vi "HAILO_Main_3d.vi"() -> ()   [LabVIEW 2016]
doc: "This example performs writes and reads on a serial port, as directed by the user. You can press the Write and Read buttons, and change the Read Count, while the example is running.\n\nThe parameters set for the serial port must match the parameters of the connected instrument or device. In this example, the Read Count parameter specifies the number of bytes that the serial port reads. If there were more bytes at the port than the specified number, those bytes would not be read. If there were less bytes at the port than the specified number, you would receive a timeout error.\n\nThis example expands upon the flow control options for XON and XOFF, allowing the user to choose those control characters. Also, the user can enable or disable a termination character. Some devices require a termination character in order to identify the end of command strings. Some devices send a termination character to signify the end of data to be read. This example shows how you can end the Read operation once a termination character is detected in the buffer and/or append a termination character at the end of the Write data."
uses:
  <vilib>/ptbypt/NI_PtbyPt.lvlib
panel:
  out "Stop 3D":bool
  out "Connection Status":u16(ring) items=["Connecting....", "BT Connected", "Disconnected"]
  in  "Tab Control":T1(tab)
  out "Channel":u16
  in  "Device Name":string="HAILO_Watch"
  in  "F Shear":dbl[](array[numeric])=[0.1, 0.1, 0.1, 0.1]
  in  "dT desired (ms)":u32=20
  in  "3d Display dT":i32=40
  in  "Enable  3D":bool
  in  "Camera Controller":enum16{"None", "Spherical", "Flying"}(ring)=enum."Spherical"
  in  "Rendering Destination":enum16{"3D Window", "3D Off"}(ring)=enum."3D Off"
  in  "3D Display":bool
  out "Sensor Output":dbl[](array[numeric])
  out "read buffer":string
  out "Sensor Nodes Returned":i32=384
  out "Sensor Readings":i16[][](array[numeric])=[[-533, -111, 239], [-402, 166, 184], [-184, 154, 29], [-106, 74, 11], [-532, -109, 246], [-398, 164, 175], [-205, 152, 32], [-119, 65, 9], [-529, -110, 242], [-408, 166, 184], [-198, 158, 27], [-108, 61, 6], [-539, -106, 240], [-407, 158, 183], [-191, 156, 28], [-113, 73, 15], [816, -260, 842], [539, 512, 512], [156, 425, 83], [13, 142, -72], [816, -262, 840], [528, 520, 512], [162, 425, 83], [13, 137, -84], [809, -260, 840], [538, 520, 504], [162, 432, 72], [13, 136, -84], [809, -260, 846], [538, 508, 512], [158, 435, 72], [19, 136, -79], [346, -168, 14], [287, -68, 19], [161, -34, 4], [70, -44, -7], [345, -191, 19], [279, -40, 8], [167, -16, 12], [72, -23, 2], [341, -190, 17], [285, -46, 9], [149, -15, 6], [54, -40, -2], [375, -201, 19], [282, -51, 10], [135, -37, 6], [81, -57, -12], [-80, -193, -48], [-73, -136, -12], [-5, -122, -31], [-19, -118, -17], [-118, -187, -48], [-73, -115, -22], [1, -113, -27], [-20, -111, -8], [-99, -184, -40], [-62, -145, -17], [0, -113, -37], [-7, -117, -15], [-126, -184, -50], [-72, -115, -14], [-4, -114, -25], [-29, -116, -14]]
  out "Packet OK?":bool=TRUE
  out "Packets Recieved":i32
  out "dT (ms)":dbl
  out "Shear Force":T2(graph)
  out "Normal Force":T3(graph)
  out "Time":u32=427420
  in  "Zero?":bool
  in  "Stop":bool
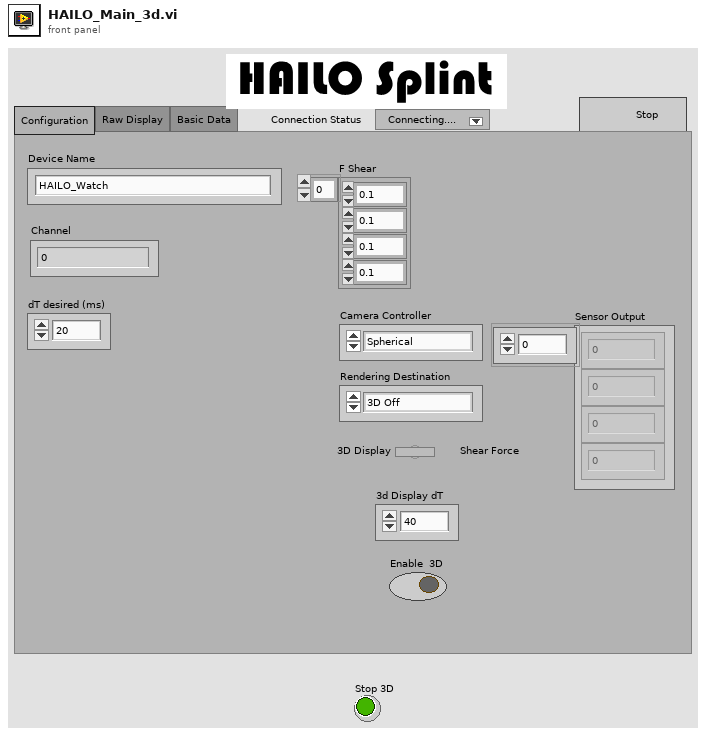
[diagram p1: front panel]
types:
  T1 = enum32{"Configuration", "Raw Display", "Basic Data"}
  T2 = cluster{"F Shear[0]":dbl, "F Shear[1]":dbl, "F Shear[2]":dbl, "F Shear[3]":dbl}
  T3 = cluster{"F Normal[0]":dbl, "F Normal[1]":dbl, "F Normal[2]":dbl, "F Normal[3]":dbl}
  T4 = cluster{"channel":u16, "uuid":string, "service name":string, "service description":string}[]
  T5 = cluster{"channel":u16, "uuid":string, "service name":string, "service description":string}
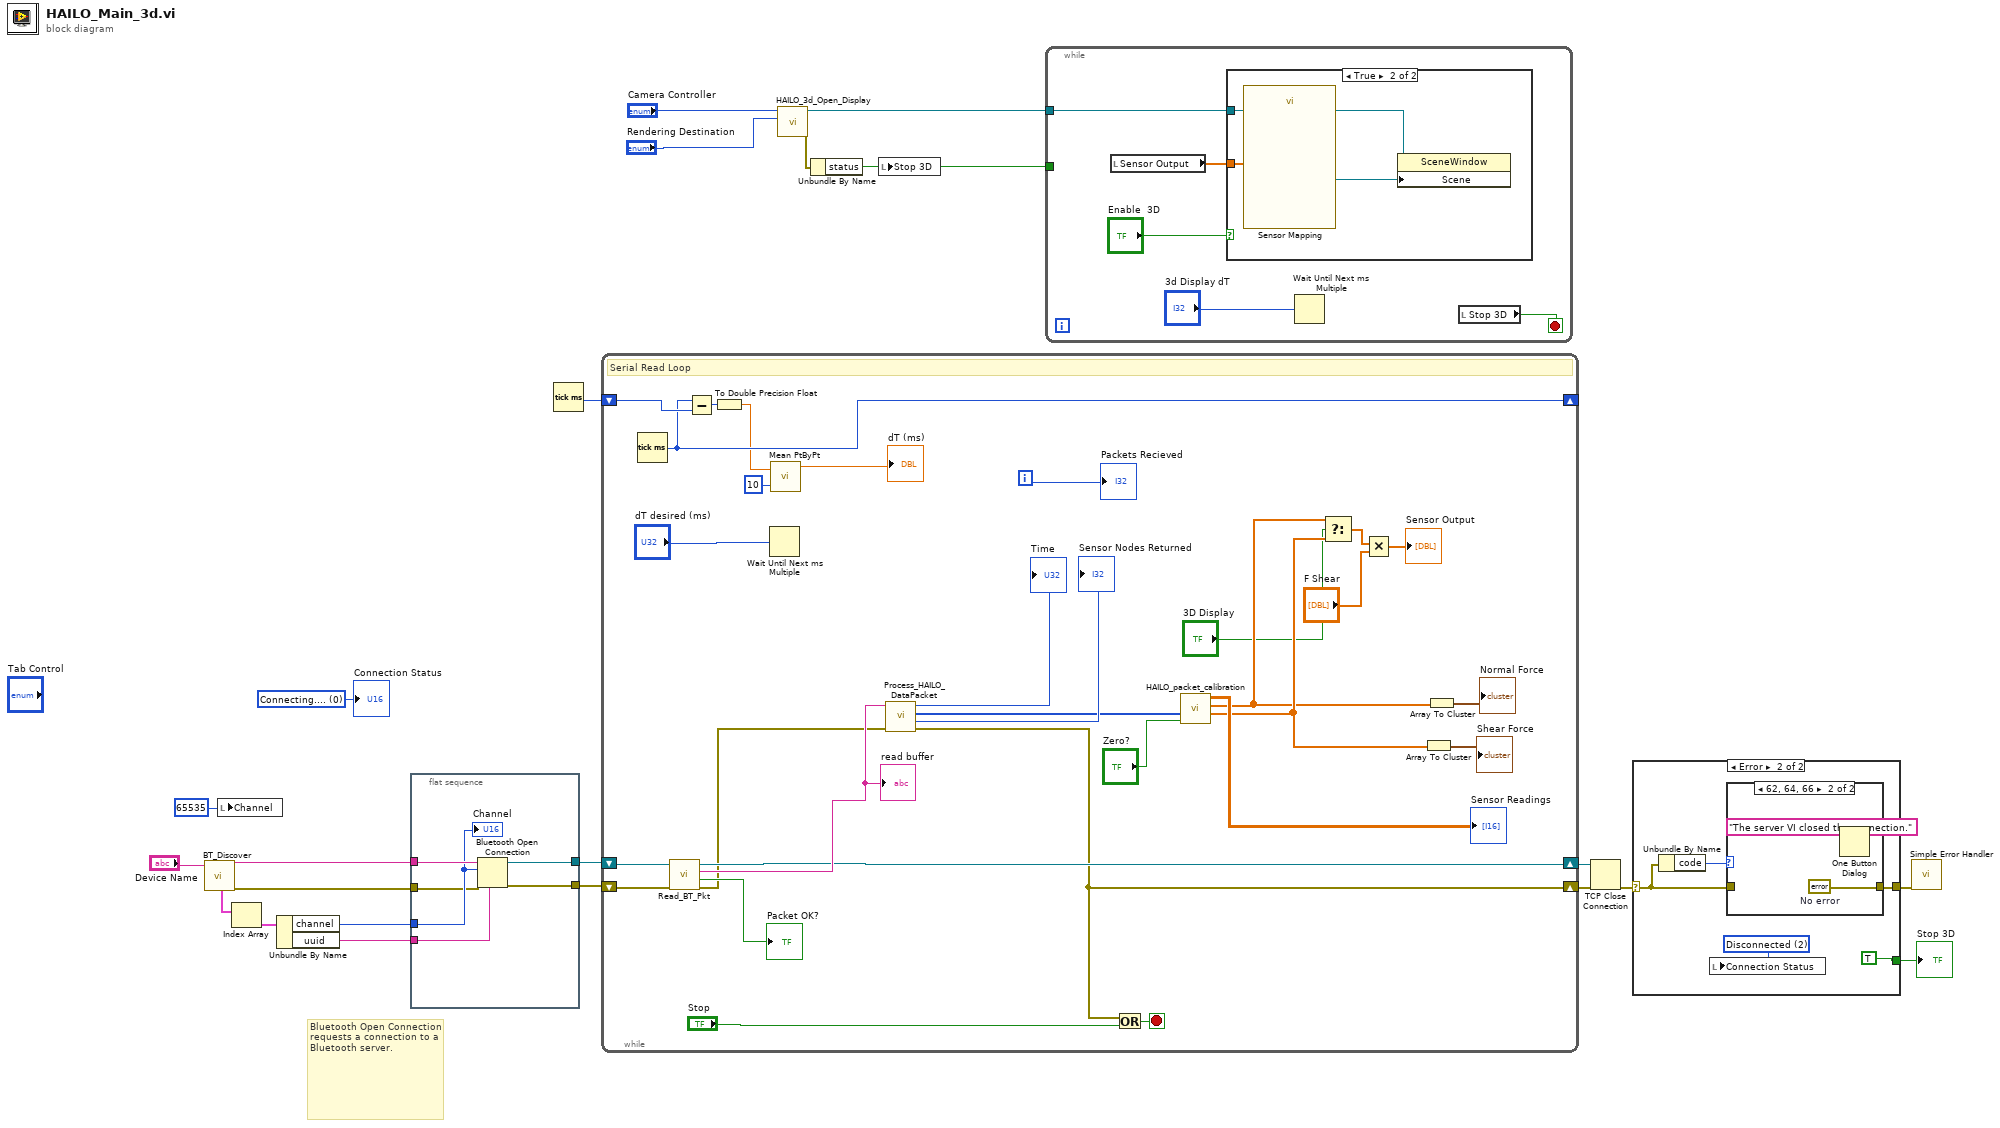
[diagram p0: block diagram]
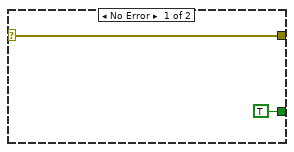
[diagram p3: hidden frame]
diagram:
  w8 = u16 0 items=["Connecting....", "BT Connected", "Disconnected"] ("Connection Status")
  # "Bluetooth Open Connection requests a connection to a Bluetooth server."
  n1 = call "BT_Discover.vi"("Device Name"="Device Name") -> ("error out"=w10:errorcluster, "Device Address"=w22:string, "service list"=w21:T4)  [unwired: 6 in, 2 out]
  n2 = local write "Channel"(u16 65535 ("Channel")) -> ()
  n3 = Index Array(array=w21) -> (element=w20:T5)  [unwired: 1 in]
  n4 = Unbundle By Name(w20) -> ("channel"=w17:u16, "uuid"=w19:string)
  n5 = flat-sequence {
    tunnel: w22 -> [w28]
    tunnel: w19 -> [w27]
    tunnel: [w26] -> w18
    tunnel: w17 -> [w25]
    tunnel: [w24] -> w15
    tunnel: w10 -> [w23]
    frame #0 {
      n6 = Bluetooth Open Connection(6:w27, 8:w23, 10:w25, 11:w28) -> (0:w24:errorcluster, 3:w26:refnum<k31>)  [unwired: 1 in]
      "Channel" <- w25
    }
  }
  n7 = Tick Count (ms)() -> (millisecond timer value=w7:u32)
  n8 = while {
    shift-right: [w51] -> w12
    shift-left: w18 -> [w55]
    shift-right: [w48] -> w11
    shift-left: w15 -> [w56]
    shift-right: [w38] -> _
    shift-left: w7 -> [w39]
    i -> [w33]
    stop <- w58 stop-if-true
    # "Serial Read Loop"
    n9 = Tick Count (ms)() -> (millisecond timer value=w38:u32)
    n10 = call "Read_BT_Pkt.vi"("error in"=w56, "connection ID in"=w55) -> ("error out"=w49:errorcluster, "Packet OK?"=→"Packet OK?":bool, "Data"=w54:string, "connection ID out"=w51:refnum<k31>)  [unwired: 6 in]
    "read buffer" <- w54
    n11 = Subtract(x=w38, y=w39) -> (x-y=w35:u32)
    n12 = To Double Precision Float(number=w35) -> (double precision float=w34:dbl)
    n13 = Wait Until Next ms Multiple(millisecond multiple="dT desired (ms)") -> ()  [unwired: 1 out]
    n14 = call <vilib>:"Mean PtByPt.vi"("x"=w34, "sample length"=10) -> ("mean"=→"dT (ms)":dbl)  [unwired: 2 in, 1 out]
    n15 = call "Process_HAILO_DataPacket.vi"("error in (no error)"=w49, "Data Packet"=w54) -> ("error out"=w48:errorcluster, "Sensor Packets Returned"=→"Sensor Nodes Returned":i32, "Sensor Readings (Signed)"=w47:i16[], "Time"=→"Time":u32)  [unwired: 6 in]
    n16 = Or(x=w48, y="Stop") -> (x .or. y?=w58:bool)
    n17 = call "HAILO_packet_calibration.vi"("Zero?"="Zero?", "Sensor Readings (Signed)"=w47) -> ("F Shear"=w41:dbl[], "F Normal"=w40:dbl[], "Sensor Readings"=→"Sensor Readings":dbl[][])  [unwired: 7 in]
    n18 = Select(t=w40, s="3D Display", f=w41) -> (s? t:f=w31:dbl[])
    n19 = Multiply(x=w31, y="F Shear") -> (x*y=→"Sensor Output":dbl[])
    n20 = Array To Cluster(array=w41) -> (cluster=→"Shear Force":T2)
    n21 = Array To Cluster(array=w40) -> (cluster=→"Normal Force":T3)
    "Packets Recieved" <- w33
  }
  n22 = call "HAILO_3d_Open_Display.vi"("Rendering Type"="Rendering Destination", "Camera Controller"="Camera Controller") -> ("error out"=w3:errorcluster, "SceneWindow out"=w2:refnum<vi>)  [unwired: 8 in]
  n23 = Unbundle By Name(w3) -> ("status"=w1:bool)
  n24 = local write "Stop 3D"(w1) -> ()
  n25 = while {
    tunnel: w2 -> [w61]
    tunnel: w1 -> [_]
    stop <- w62 stop-if-true
    n26 = local read "Sensor Output"() -> (w63:dbl[])
    n27 = case shown="True" "Enable  3D" {
      tunnel: w63 -> [_ w66]
      tunnel: w61 -> [_ w65]
      frame False {
      }
      frame True {
        n28 = call "Sensor Mapping"("Sensor Values"=w66) -> ("Scene Ref Out"=w64:refnum<vi>)  [unwired: 9 in, 1 out]
        n29 = property class="SceneWindow"(reference=w65, "Scene"=w64) -> ()  [unwired: 1 in, 2 out]
      }
    }
    n30 = Wait Until Next ms Multiple(millisecond multiple="3d Display dT") -> ()  [unwired: 1 out]
    n31 = local read "Stop 3D"() -> (w62:bool)
  }
  n32 = TCP Close Connection(connection ID=w12, error in (no error)=w11) -> (error out=w14:errorcluster)  [unwired: 1 in, 1 out]
  n33 = case shown="Error" w14 {
    selector: w14 -> [w68 w72]
    tunnel: [w68 w71] -> w13
    tunnel: [TRUE TRUE] -> w4
    frame No Error {
    }
    frame Error {
      w70 = u16 2 items=["Connecting....", "BT Connected", "Disconnected"] ("Connection Status")
      n34 = Unbundle By Name(w72) -> ("code"=w73:i32)
      n35 = local write "Connection Status"(w70) -> ()
      n36 = case shown="62, 64, 66" w73 {
        tunnel: w72 -> [w74 _]
        tunnel: [w74 w76] -> w71
        frame Default {
        }
        frame 62, 64, 66 {
          w76 = errorcluster {"status"=FALSE, "code"=0, "source"=""}  # No error
          n37 = One Button Dialog(message="The server VI closed the connection." ("Server Closed")) -> ()  [unwired: 1 in, 1 out]
        }
      }
    }
  }
  "Stop 3D" <- w4
  n38 = call <vilib>:"Simple Error Handler.vi"("error in (no error)"=w13) -> ()  [unwired: 4 in, 5 out]
  "Connection Status" <- w8
